vi "Get Parent Class.vi"(8 "error in (no error)":errorcluster, 10 "Test Class Path":path) -> (0 "error out":errorcluster, 2 "Path":path)   [LabVIEW 2020, in "Pure Mock Class Generator Test.lvclass"]
uses:
  Pure Mock Class Generator Test.lvclass
  Pure Mock Class Generator Test.lvclass/Pure Mock Class Generator Test.ctl
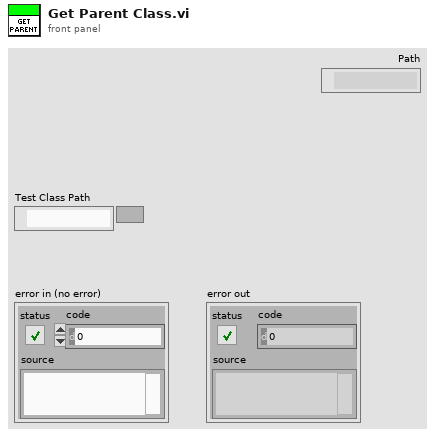
[diagram p1: front panel]
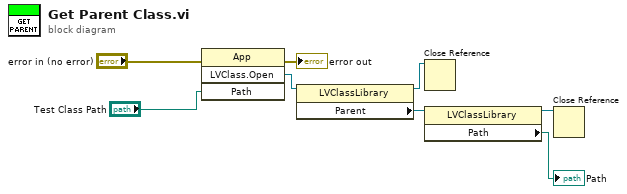
[diagram p0: block diagram]
diagram:
  n1 = invoke class="App" method="LVClass.Open"(error in="error in (no error)", "Path"="Test Class Path") -> (error out=→"error out":errorcluster, "LVClass.Open"=w5:refnum<vi>)  [unwired: 2 in, 2 out]
  n2 = property class="LVClassLibrary"(reference=w5) -> (reference out=w2:refnum<vi>, "Parent"=w4:refnum<vi>)  [unwired: 1 in, 1 out]
  n3 = Close Reference(reference=w2) -> ()  [unwired: 1 in, 1 out]
  n4 = property class="LVClassLibrary"(reference=w4) -> (reference out=w1:refnum<vi>, "Path"=→"Path":path)  [unwired: 1 in, 1 out]
  n5 = Close Reference(reference=w1) -> ()  [unwired: 1 in, 1 out]
